vi "Stepper SM Check State.vi"(1 "State in":T1) -> (0 "State out":T1)   [LabVIEW 2015]
uses:
  Controls/Stepper SM Enumerator.ctl
  <vilib>/rvi/eio/common/nirviEmuTemplateMethod_errors.vi
  <vilib>/eio/EIOMethodNode/EIOMethodNode.xnode
  <vilib>/LabVIEW Targets/FPGA/cRIO/shared/nicrio_ModuleControls/nicrio_cRIO-950x_DriveStatus.ctl
  <vilib>/eio/EIONode/EIONode.xnode
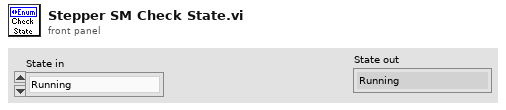
[diagram p1: front panel]
types:
  T1 = typedef "Stepper SM Enumerator.ctl" = enum16{"Running", "Backing up", "Idle", "Home", "Lim"}
  T2 = typedef "nicrio_cRIO-950x_DriveStatus.ctl" = enum8{"Drive Disabled (Rated phase current set to zero)", "Drive Disabled (Disabled by fault)", "Drive Disabled (Disabled by software)", "Drive Enabled"}
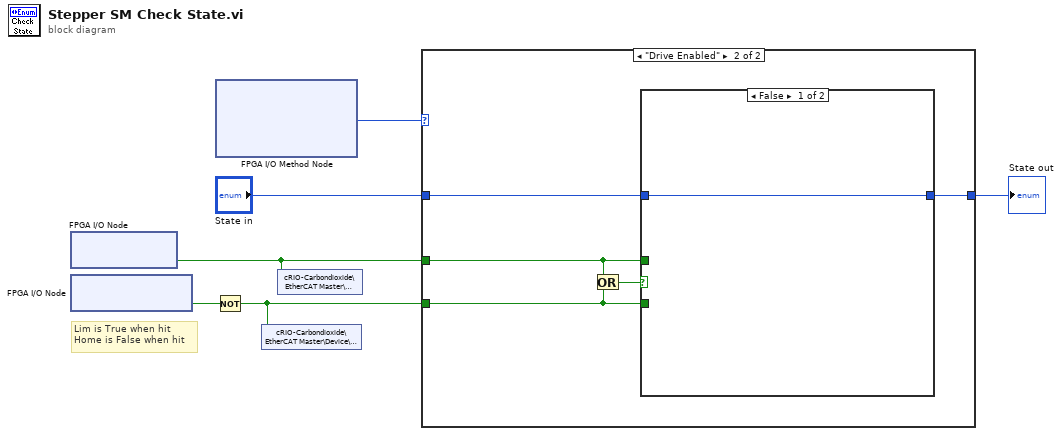
[diagram p0: block diagram]
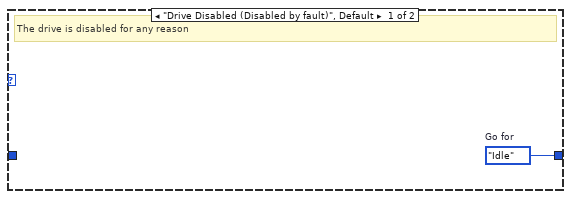
[diagram p2: hidden frame]
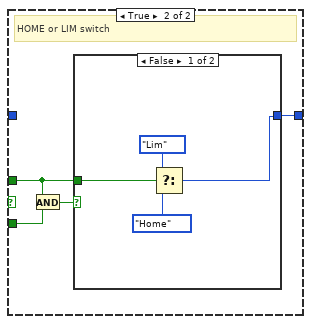
[diagram p3: hidden frame]
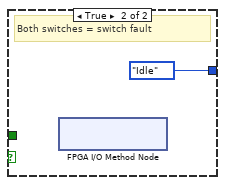
[diagram p4: hidden frame]
diagram:
  # "Lim is True when hit\nHome is False when hit"
  n1 = xnode "FPGA I/O Node"() -> ("Stepper LIM"=w1:bool)  [unwired: 1 in, 1 out]
  n2 = xnode "FPGA I/O Node"() -> ("Stepper HOME"=w3:bool)  [unwired: 1 in, 1 out]
  n3 = Not(x=w3) -> (.not. x?=w2:bool)
  n4 = xnode "FPGA I/O Method Node"() -> ("Drive Status"=w4:T2)  [unwired: 1 in, 3 out]
  n5 = shared-variable "cRIO-Carbondioxide\\EtherCAT Master\\Device\\User-Defined Variables\\SM HOME"(w2) -> ()  [unwired: 1 in, 1 out]
  n6 = shared-variable "cRIO-Carbondioxide\\EtherCAT Master\\Device\\User-Defined Variables\\SM LIM"(w1) -> ()  [unwired: 1 in, 1 out]
  n7 = case shown="\"Drive Enabled\"" w4 {
    tunnel: "State in" -> [_ w11]
    tunnel: [w7 w10] -> w5
    tunnel: w1 -> [_ w9]
    tunnel: w2 -> [_ w8]
    frame "Drive Disabled (Disabled by fault)", Default {
      w7 = Stepper_SM_Enumerator."Idle"  # Go for
      # "The drive is disabled for any reason"
    }
    frame "Drive Enabled" {
      n8 = Or(x=w9, y=w8) -> (x .or. y?=w12:bool)
      n9 = case shown="False" w12 {
        tunnel: w11 -> [w13 _]
        tunnel: w9 -> [_ w15]
        tunnel: w8 -> [_ w14]
        tunnel: [w13 w16] -> w10
        frame False {
        }
        frame True {
          # "HOME or LIM switch"
          n10 = And(x=w15, y=w14) -> (x .and. y?=w17:bool)
          n11 = case shown="False" w17 {
            tunnel: [w18 Stepper_SM_Enumerator."Idle" ("State in")] -> w16
            tunnel: w15 -> [w21 _]
            frame False {
              n12 = Select(t=Stepper_SM_Enumerator."Lim" ("State in"), s=w21, f=Stepper_SM_Enumerator."Home") -> (s? t:f=w18:T1)
            }
            frame True {
              # "Both switches = switch fault"
              n13 = xnode "FPGA I/O Method Node"() -> ()  [unwired: 1 in, 1 out]
            }
          }
        }
      }
    }
  }
  "State out" <- w5
